vi "UI.vi"   [LabVIEW 2014]
uses:
  <vilib>/rvi/interface/RandomDataEmulation/nirviRandomDataOpen.vi
  <vilib>/rvi/interface/common/niFpgaCacheSessionInfoDynamic.vi
  <vilib>/rvi/interface/nirviOpenFPGA/nirviOpenFPGA.xnode
  Top Level FPGA.vi
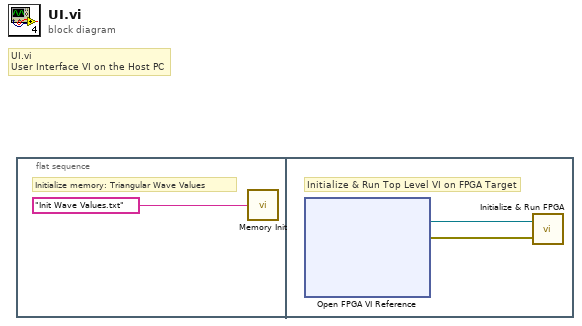
[diagram p0: block diagram]
diagram:
  # "UI.vi\nUser Interface VI on the Host PC"
  n1 = flat-sequence {
    frame #0 {
      # "Initialize memory: Triangular Wave Values"
      n2 = call "Memory Init.vi"("File name"="Init Wave Values.txt" ("name or relative path")) -> ()  [unwired: 1 in]
    }
    frame #1 {
      # "Initialize & Run Top Level VI on FPGA Target"
      n3 = xnode "Open FPGA VI Reference"() -> ("FPGA VI Reference Out"=w3:refnum<k20>, "error out"=w2:errorcluster)  [unwired: 2 in]
      n4 = call "Initialize & Run FPGA.vi"("error in"=w2, "FPGA VI Reference In"=w3) -> ()  [unwired: 2 out]
    }
  }
